vi "Init.vi"(8 "error in (no error)":errorcluster, 10 "Instrument String":variant, 11 "KEithley 27XX DMM in":refnum<class "Keithley 27XX DMM.lvclass">) -> (0 "error out":errorcluster, 2 "Found?":bool, 3 "KEithley 27XX  DMM out":refnum<class "Keithley 27XX DMM.lvclass">)   [LabVIEW 2025, in "DMM.lvlib" / "Keithley 27XX DMM.lvclass"]
uses:
  Keithley 27XX DMM.lvclass
  C:/Working copy/tss/Plugin/Engines/DMM/DMM Instrument/DMM Instrument.lvclass
  DMM configuration/DMM configuration.lvclass
  C:/Users/Public/Documents/Sandia National Labs/TSS Plugin/Abstract Engine.lvlibp/Plugin/Abstract/Instrument configuration/Instrument configuration.lvclass
  Keithley 27XX DMM.lvclass/Keithley 27XX DMM.ctl
  Users/Public/Documents/Sandia National Labs/TSS Plugin/Abstract Engine.lvlibp/Plugin/Abstract/Instrument configuration/Read Instrument Setting.vi
  Users/Public/Documents/Sandia National Labs/TSS Plugin/CEF.lvlibp/serializable configuration/CEF_serializable configuration.lvclass
  <instrlib>/Keithley 27XX/Keithley 27XX.lvlib
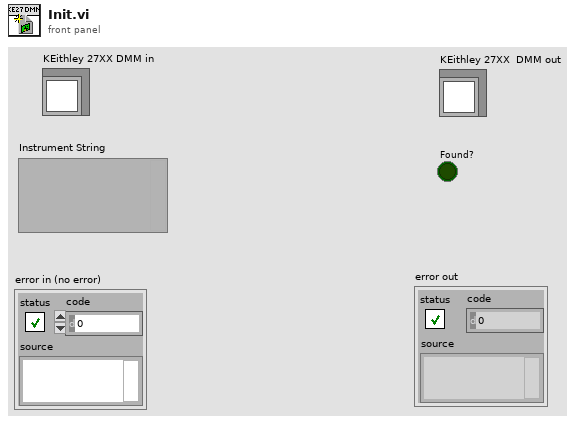
[diagram p1: front panel]
types:
  T1 = typedef "Abstract Engine.lvlibp/Instrument configuration.lvclass/Default Instrument.ctl" = cluster{"Type":string, "Address":string, "SW Alias":string, "Description":string, "Enabled":bool}
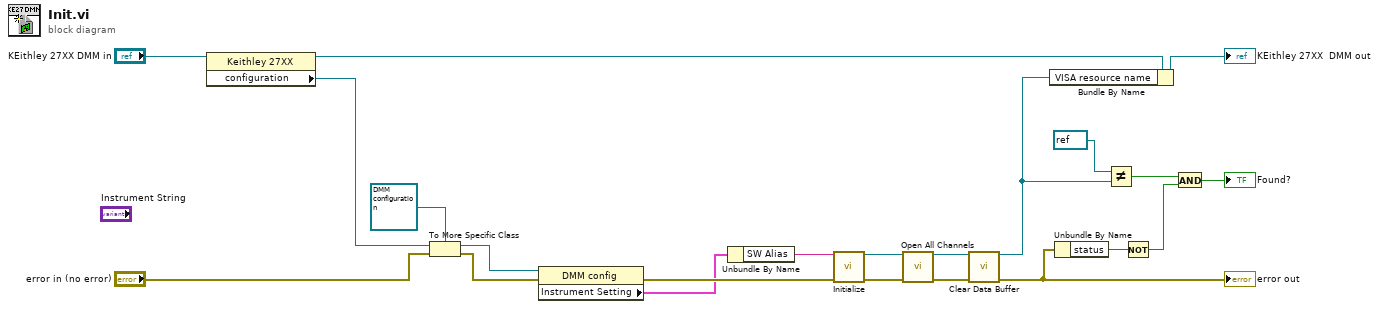
[diagram p0: block diagram]
diagram:
  n1 = property class="Keithley 27XX"(reference="KEithley 27XX DMM in") -> (reference out=w10:refnum<class "Keithley 27XX DMM.lvclass">, "configuration"=w17:refnum<class "CEF_serializable configuration.lvclass">)  [unwired: 1 in, 1 out]
  n2 = To More Specific Class(target class=refnum<class "DMM configuration.lvclass"> refnum ("DMM.lvlib:DMM configuration.lvclass"), reference=w17, error in="error in (no error)") -> (specific class reference=w16:refnum<class "DMM configuration.lvclass">, error out=w15:errorcluster)
  n3 = property class="DMM config"(reference=w16, error in=w15) -> (error out=w13:errorcluster, "Instrument Setting"=w1:T1)  [unwired: 1 out]
  n4 = Unbundle By Name(w1) -> ("SW Alias"=w12:string)
  n5 = call <instrlib>:"Initialize.vi"("VISA resource name"=w12, "error in (no error)"=w13) -> ("VISA resource name out"=w21:refnum<visa-resource-name>, "error out"=w22:errorcluster)  [unwired: 12 in]
  n6 = call <instrlib>:"Open All Channels.vi"("VISA resource name"=w21, "error in (no error)"=w22) -> ("VISA resource name out"=w19:refnum<visa-resource-name>, "error out"=w20:errorcluster)  [unwired: 12 in]
  n7 = call <instrlib>:"Clear Data Buffer.vi"("VISA resource name"=w19, "error in (no error)"=w20) -> ("VISA resource name out"=w8:refnum<visa-resource-name>, "error out"=w5:errorcluster)  [unwired: 12 in]
  "error out" <- w5
  n8 = Bundle By Name(cluster=w10, "VISA resource name"=w8) -> (→"KEithley 27XX  DMM out":refnum<class "Keithley 27XX DMM.lvclass">)
  n9 = Unbundle By Name(w5) -> ("status"=w6:bool)
  n10 = Not Equal?(x=refnum<visa-resource-name> refnum ("VISA resource name out"), y=w8) -> (x != y?=w4:bool)
  n11 = Not(x=w6) -> (.not. x?=w3:bool)
  n12 = And(x=w4, y=w3) -> (x .and. y?=→"Found?":bool)
